vi "SV Get By Measurement Type (sw trigger) (1 Ch).vi"(0 "scaled signals [EU]":waveform(dbl)[](array[waveform])) -> (4 "scaled signals with trigger channel deleted":waveform(dbl)[](array[waveform]), 6 "found?":bool, 8 "trigger channel":waveform(dbl), 10 "trigger index":i32, 12 "trigger channel name":string, 13 "pretrigger samples":i32, 14 "level trigger configuration":T1={"level"=0.0, "slope"=1, "hysteresis"=0.0} {"hysteresis" format="%.2p"; "slope" items=["Falling Edge", "Rising Edge"]; "level" format="%.2p"})   [LabVIEW 2017]
doc: "Separates data from an array of waveforms based on the type of measurement selected. This VI requires that waveform attributes such as NI_UnitDescription are added by NI DAQmx."
uses:
  <vilib>/addons/_NISVFA/_Shared subVIs/Common/sv_Get SV Property Name String.vi
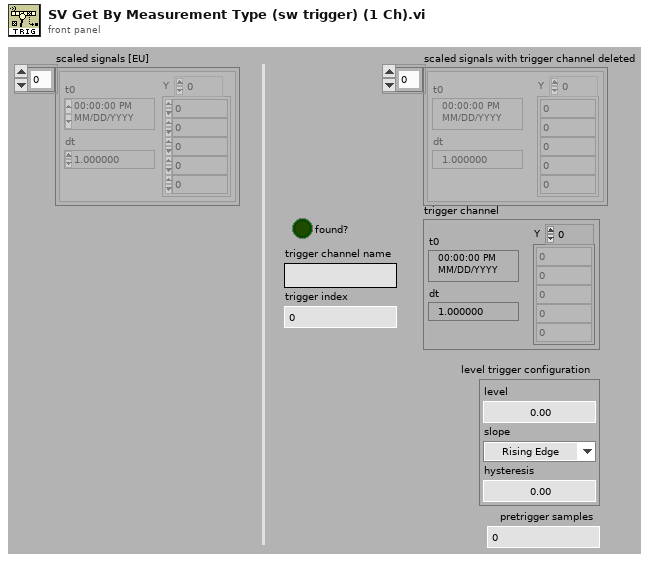
[diagram p1: front panel]
types:
  T1 = cluster{"level":dbl, "slope":u16, "hysteresis":dbl}
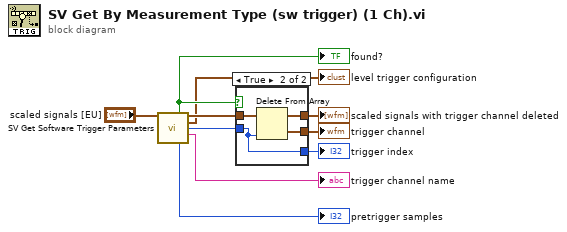
[diagram p0: block diagram]
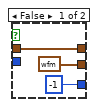
[diagram p2: hidden frame]
diagram:
  n1 = call <vilib>:"SV Get Software Trigger Parameters.vi"("scaled signals [EU] in"="scaled signals [EU]") -> ("trigger channel found"=w4:bool, "scaled signals [EU] out"=w7:waveform(dbl)[], "level trigger configuration"=→"level trigger configuration":T1, "trigger index"=w3:i32, "trigger channel name"=→"trigger channel name":string, "pretrigger samples"=→"pretrigger samples":i32)  [unwired: 7 in, 2 out]
  "found?" <- w4
  n2 = case shown="True" w4 {
    tunnel: [w11 w17] -> w6
    tunnel: [waveform(dbl) {"t0"=timestamp(0 s since 1904-01-01), "dt"=1.0, "Y"=[]} ("Waveform") w14] -> w10
    tunnel: [-1 w15] -> w9
    tunnel: w7 -> [w11 w16]
    tunnel: w3 -> [_ w15]
    frame False {
    }
    frame True {
      n3 = Delete From Array(array=w16, index=w15) -> (deleted portion=w14:waveform(dbl), array with subset deleted=w17:waveform(dbl)[])  [unwired: 1 in]
    }
  }
  "trigger channel" <- w10
  "scaled signals with trigger channel deleted" <- w6
  "trigger index" <- w9
